vi "ventoinha com switch case.vi"() -> ()   [LabVIEW 2018]
panel:
  out "Fan is ON":bool
  in  "stop":bool
  out "Thermometer":dbl(slide) scale=0.0..100.0
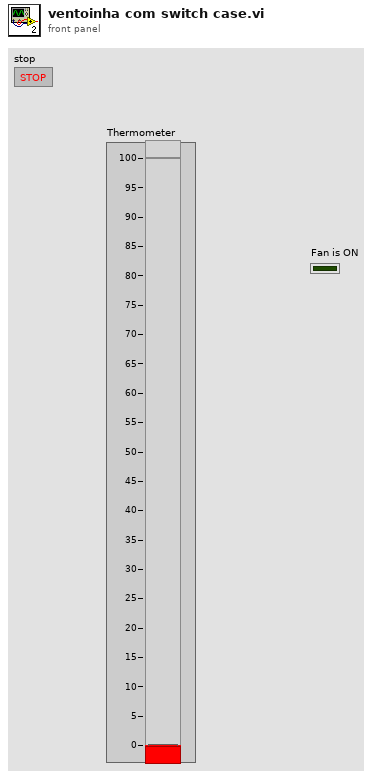
[diagram p1: front panel]
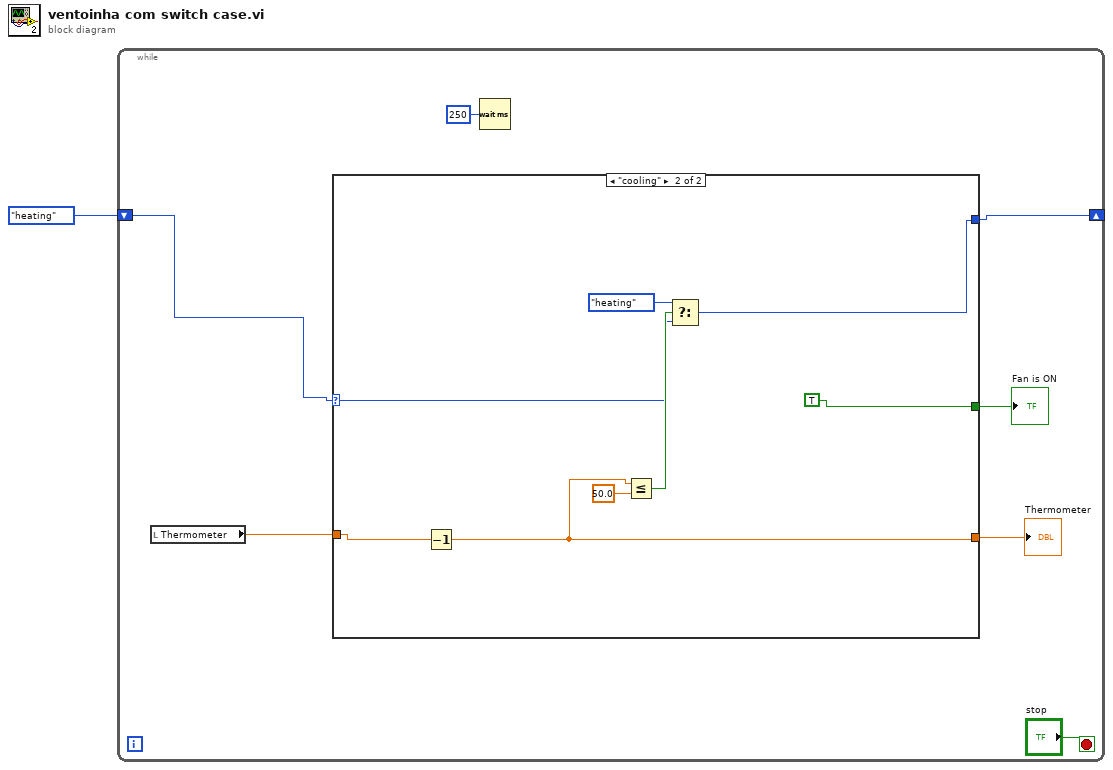
[diagram p0: block diagram]
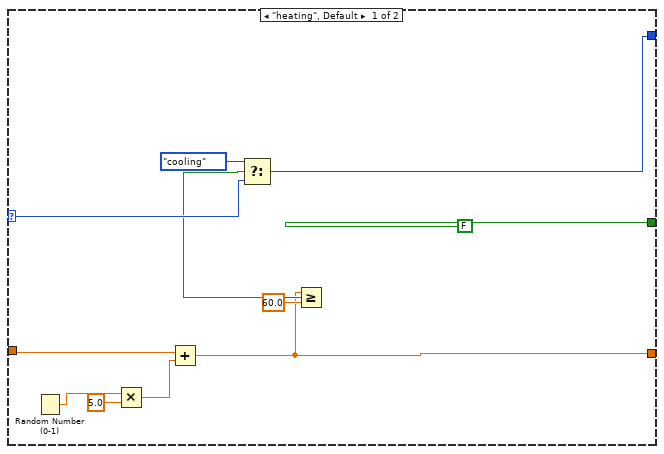
[diagram p2: hidden frame]
diagram:
  n1 = while {
    shift-right: [w7] -> _
    shift-left: enum16{"heating", "cooling"}."heating" -> [w8]
    stop <- "stop" stop-if-true
    n2 = local read "Thermometer"() -> (w6:dbl)
    n3 = case shown="\"cooling\"" w8 {
      selector: w8 -> [w19 w21]
      tunnel: [w10 w27] -> w7
      tunnel: w6 -> [w14 w25]
      tunnel: [w11 w23] -> w5
      tunnel: [FALSE TRUE] -> w2
      frame "heating", Default {
        n4 = Random Number (0-1)() -> (number: 0 to 1=w18:dbl)
        n5 = Multiply(x=w18, y=5.0) -> (x*y=w16:dbl)
        n6 = Add(x=w14, y=w16) -> (x+y=w11:dbl)
        n7 = Greater Or Equal?(x=w11, y=60.0) -> (x >= y?=w13:bool)
        n8 = Select(t=enum16{"heating", "cooling"}."cooling", s=w13, f=w19) -> (s? t:f=w10:enum16{"heating", "cooling"})
      }
      frame "cooling" {
        n9 = Decrement(x=w25) -> (x-1=w23:dbl)
        n10 = Less Or Equal?(x=w23, y=50.0) -> (x <= y?=w22:bool)
        n11 = Select(t=enum16{"heating", "cooling"}."heating", s=w22, f=w21) -> (s? t:f=w27:enum16{"heating", "cooling"})
      }
    }
    "Thermometer" <- w5
    "Fan is ON" <- w2
    n12 = Wait (ms)(milliseconds to wait=u32 250) -> ()  [unwired: 1 out]
  }
